vi "ArrayColorRgbaU32ToImage.vi"(8 "error in":errorcluster, 10 "Pixel":T1[][](array[typedef]), 11 "Image Reference In":T2) -> (0 "error out":errorcluster, 3 "Image Reference Out":T2)   [LabVIEW 2024, in "OpenLvVision_Image.lvlib" / "DataAccess.lvlib"]
doc: "Replaces the image's data with the provided array (Copy)"
uses:
  Management/TypeDef/Image.ctl
  TypeDef/RgbaU32.ctl
  DataAccess.lvlib
  Management/Management.lvlib
  TypeDef/StepSizes.ctl
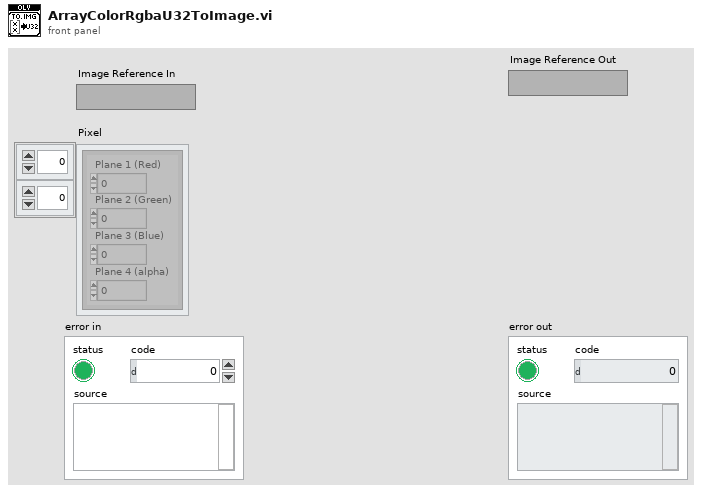
[diagram p1: front panel]
types:
  T1 = typedef "OpenLvVision_Image.lvlib/DataAccess.lvlib/RgbaU32.ctl" = cluster{"Plane 1 (Red)":u8, "Plane 2 (Green)":u8, "Plane 3 (Blue)":u8, "Plane 4 (alpha)":u8}
  T2 = typedef "OpenLvVision_Image.lvlib/Management.lvlib/Image.ctl" = refnum<image>
  T3 = typedef "OpenLvVision_Image.lvlib/DataAccess.lvlib/StepSizes.ctl" = cluster{"X Step Size":u32, "Y Step Size":u32}
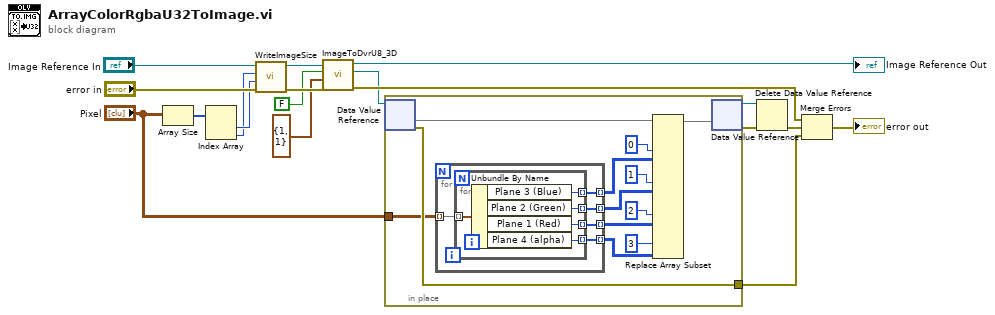
[diagram p0: block diagram]
diagram:
  n1 = Array Size(array="Pixel") -> (size(s)=w15:i32[])
  n2 = Index Array(array=w15) -> (element #1=w14:i32, element #2=w13:i32)  [unwired: 2 in]
  n3 = call "WriteImageSize.vi"("error in"="error in", "Height"=w14, "Width"=w13, "Image Reference In"="Image Reference In") -> ("error out"=w11:errorcluster, "Image Reference Out"=w12:T2)  [unwired: 6 in]
  n4 = call "ImageToDvrU8_3D.vi"("error in"=w11, "Step Sizes"=T3 {"X Step Size"=1, "Y Step Size"=1}, "Include Border"=FALSE, "Image Reference In"=w12) -> ("error out"=w4:errorcluster, "EDVR 3D U8"=w3:refnum<data-value>, "Image Reference Out"=→"Image Reference Out":T2)  [unwired: 4 in, 1 out]
  n5 = in-place {
    in-place-border: "Pixel" -> [w19]
    in-place-border: [w20] -> w5
    n6 = in-place-dvr #1(w3) -> (w30:u8[][][], w20:errorcluster)
    n7 = for {
      tunnel: w19 -> [w35] mode=indexing
      tunnel: [w34] -> w28 mode=indexing
      tunnel: [w33] -> w26 mode=indexing
      tunnel: [w32] -> w25 mode=indexing
      tunnel: [w31] -> w24 mode=indexing
      n8 = for {
        tunnel: w35 -> [w40] mode=indexing
        tunnel: [w39] -> w34 mode=indexing
        tunnel: [w38] -> w33 mode=indexing
        tunnel: [w37] -> w32 mode=indexing
        tunnel: [w36] -> w31 mode=indexing
        n9 = Unbundle By Name(w40) -> ("Plane 3 (Blue)"=w39:u8, "Plane 2 (Green)"=w38:u8, "Plane 1 (Red)"=w37:u8, "Plane 4 (alpha)"=w36:u8)
      }
    }
    n10 = Replace Array Subset(array=w30, new element #1=w28, index (dim 2) #1=0 ("disabled index (col)"), new element #2=w26, index (dim 2) #2=1 ("disabled index (col)"), new element #3=w25, index (dim 2) #3=2 ("disabled index (col)"), new element #4=w24, index (dim 2) #4=3 ("disabled index (col)")) -> (w29:u8[][][])  [unwired: 8 in]
    n11 = in-place-dvr #1(w29) -> (w9:refnum<data-value>, w8:errorcluster)
  }
  n12 = Delete Data Value Reference(data value reference=w9, error in=w8) -> (error out=w7:errorcluster)  [unwired: 1 out]
  n13 = Merge Errors(w4, w7, w5) -> (→"error out":errorcluster)
